vi "Jacobian.vi"(10 "EE Position":dbl[](array[numeric]), 11 "Motor Configuration":dbl[][](array[numeric])) -> (3 "Jacobian":T1)   [LabVIEW 2021]
uses:
  <vilib>/Analysis/Matrix/Datatypes/RealMatrix.ctl
  <vilib>/Analysis/_algsub.llb/Real Vector Norm.vi
  <vilib>/Analysis/Matrix/Numeric/Conversions/Array To Matrix - RA2.vi
  <vilib>/Analysis/NI_AALPro.lvlib
  <vilib>/Analysis/Matrix/NI_Matrix.lvlib
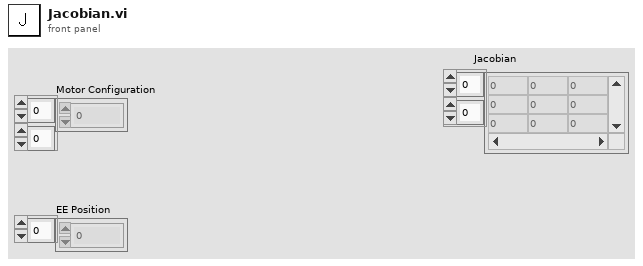
[diagram p1: front panel]
types:
  T1 = typedef "NI_Matrix.lvlib/RealMatrix.ctl" = dbl[][]
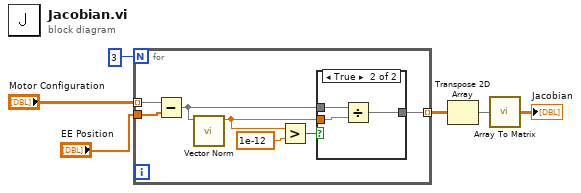
[diagram p0: block diagram]
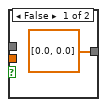
[diagram p2: hidden frame]
diagram:
  n1 = for {
    N: 3 -> [_]
    tunnel: "Motor Configuration" -> [w7] mode=indexing
    tunnel: "EE Position" -> [w9]
    tunnel: [w8] -> w3 mode=indexing
    n2 = Subtract(x=w7, y=w9) -> (x-y=w12:dbl[])
    n3 = call-poly <vilib>:"Vector Norm.vi"("Input Vector"=w12) -> ("norm"=w13:dbl)  [unwired: 9 in, 1 out]
    n4 = Greater?(x=w13, y=1e-12) -> (0:w11:bool)
    n5 = case shown="True" w11 {
      tunnel: w12 -> [_ w17]
      tunnel: w13 -> [_ w16]
      tunnel: [dbl[] [0.0, 0.0] w15] -> w8
      frame False {
      }
      frame True {
        n6 = Divide(x=w17, y=w16) -> (x/y=w15:dbl[])
      }
    }
  }
  n7 = Transpose 2D Array(2D array=w3) -> (transposed array=w2:dbl[][])
  n8 = call-poly <vilib>:"Array To Matrix.vi"("Real 2D Array"=w2) -> ("Real Matrix"=→"Jacobian":T1)
